vi "RSZVB Set Source Power Calibration Sensitivity Correction Range.vi"(8 "error in (no error)":errorcluster {"code" format="%.0x"}, 9 "Frequency Range (From Power Meter Entry In Port Configuration)":i32(ring)=1 items=["From Source To Be Calibrated", "From Power Meter Entry In Port Configuration"], 10 "Channel (1)":i32=1, 11 "VISA session":refnum<visa-resource-name>) -> (0 "error out":errorcluster {"code" format="%.0x"}, 3 "dup VISA session":refnum<visa-resource-name>)   [LabVIEW 2011]
doc: "Selects the frequency range for the sensitivity correction of the power meter.\n\nRemote-control command(s):\n[SENSe<Ch>:]PMMO ON | OFF"
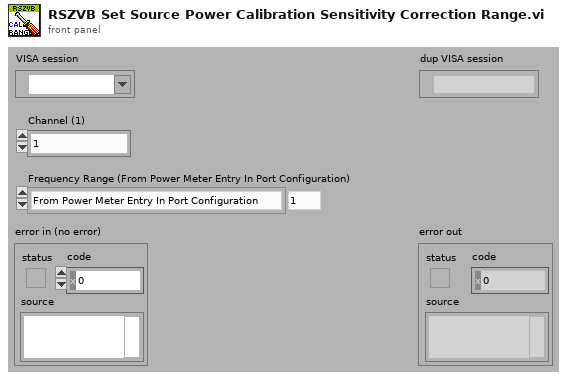
[diagram p1: front panel]
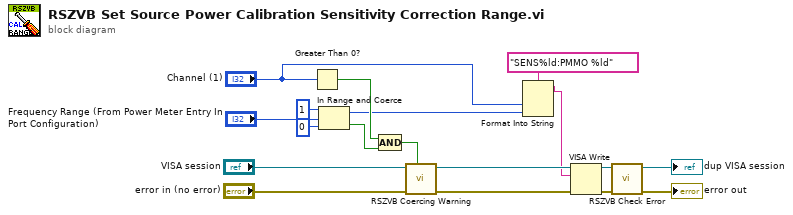
[diagram p0: block diagram]
diagram:
  n1 = Greater Than 0?(x="Channel (1)") -> (x > 0?=w10:bool)
  n2 = In Range and Coerce(upper limit=1, x="Frequency Range (From Power Meter Entry In Port Configuration)", lower limit=0) -> (coerced(x)=w1:i32, In Range?=w9:bool)
  n3 = Compound Arithmetic op=AND(w10, w9) -> (w8:bool)
  n4 = call "RSZVB Coercing Warning.vi"("In Range?"=w8, "error in (no error)"="error in (no error)", "VISA session"="VISA session") -> ("error out"=w17:errorcluster, "dup VISA session"=w18:refnum<visa-resource-name>)  [unwired: 7 in]
  n5 = Format Into String(format string="SENS%ld:PMMO %ld", "Channel (1)", w1) -> (resulting string=w13:string)  [unwired: 2 in, 1 out]
  n6 = VISA Write(VISA resource name=w18, write buffer=w13, error in (no error)=w17) -> (VISA resource name out=w15:refnum<visa-resource-name>, error out=w16:errorcluster)  [unwired: 1 out]
  n7 = call "RSZVB Check Error.vi"("error in (no error)"=w16, "VISA session"=w15) -> ("error out"=→"error out":errorcluster, "dup VISA session"=→"dup VISA session":refnum<visa-resource-name>)  [unwired: 8 in]
